vi "Update Slot Name.vi"(8 "error in":errorcluster, 10 "module":T1, 11 "slot ref in":T2 format="%.0x") -> (0 "error out":errorcluster, 2 "name":string, 3 "slot ref out":T2 format="%.0x")   [LabVIEW 2020, in "SEECD System Explorer.lvlib"]
uses:
  SEECD System Explorer.lvlib
  <vilib>/NI VeriStand/Custom Device API/Custom Device Item Ref.ctl
  Includes/Modules.lvlibp/RSI Module/Module Models.ctl
  <vilib>/dlg_ctls.llb/Space Constant.vi
  Shared/SEECD Shared.lvlib
  <vilib>/NI VeriStand/Custom Device API/Custom Device API.lvlib
  Includes/Modules.lvlibp/RSI Module/RSI Module.lvclass
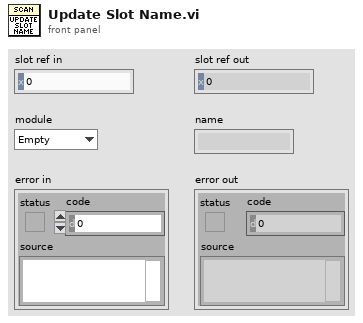
[diagram p1: front panel]
types:
  T1 = typedef "Modules.lvlibp/RSI Module.lvclass/Module Models.ctl" = enum16{"Empty", "NI 9201", "NI 9203", "NI 9205", "NI 9206", "NI 9207", "NI 9208", "NI 9209", "NI 9210", "NI 9211", "NI 9212", "NI 9213", "NI 9214", "NI 9215", "NI 9216", "NI 9217", "NI 9219", "NI 9220", "NI 9221", "NI 9222", "NI 9223", "NI 9224", "NI 9225", "NI 9226", "NI 9227", "NI 9228", "NI 9229", "NI 9233", "NI 9234", "NI 9235", "NI 9236", "NI 9237", "NI 9239", "NI 9242", "NI 9244", "NI 9253", "NI 9263", "NI 9264", "NI 9265", "NI 9266", "NI 9269", "NI 9344", "NI 9350", "NI 9375", "NI 9401", "NI 9402", "NI 9403", "NI 9411", "NI 9421", "NI 9422", "NI 9423", "NI 9425", "NI 9426", "NI 9435", "NI 9436", "NI 9437", "NI 9472", "NI 9474", "NI 9475", "NI 9476", "NI 9477", "NI 9478", "NI 9481", "NI 9482", "NI 9485"}
  T2 = typedef "Custom Device API.lvlib/Custom Device Item Ref.ctl" = u64
  T3 = typedef "Custom Device API.lvlib/Custom Device Item Info.ctl" = cluster{"Name":string, "Is Channel":bool, "GUID":string, "Is Waveform":bool}
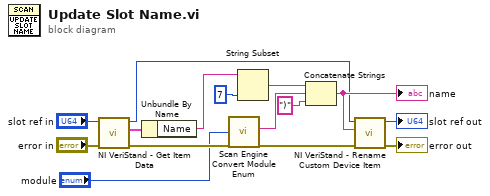
[diagram p0: block diagram]
diagram:
  n1 = call <vilib>:"NI VeriStand - Get Item Data.vi"("error in (no error)"="error in", "Item Ref in"="slot ref in") -> ("error out"=w3:errorcluster, "Item Info"=w5:T3, "Item Ref out"=w2:T2)  [unwired: 6 in, 1 out]
  n2 = Unbundle By Name(w5) -> ("Name"=w4:string)
  n3 = call "Scan Engine Convert Module Enum.vi"("Module"="module") -> ("Module Name"=w14:string)  [unwired: 2 in, 1 out]
  n4 = String Subset(string=w4, length (rest)=7 ("length (rest)")) -> (substring=w12:string)  [unwired: 1 in]
  n5 = Concatenate Strings(w12, w14, ")" ("string")) -> (w10:string)
  "name" <- w10
  n6 = call <vilib>:"NI VeriStand - Rename Custom Device Item.vi"("error in (no error)"=w3, "New Name"=w10, "Item Ref in"=w2) -> ("error out"=→"error out":errorcluster, "Item Ref out"=→"slot ref out":T2)  [unwired: 1 in, 6 out]
